vi "wavedump.vi"() -> ()   [LabVIEW 2018]
panel:
  in  "Plot":bool
  in  "?":enum32{"Output", "README"}(tab)
  out "Command Line Output":string
  in  "Stop":bool
  in  "Start":bool
  in  "Run":bool
  in  "Write":bool
  in  "Close":bool
  # "This vi is used to send wavedump commands.\n\nRun to run wavedump\n\nStart to start data aquisition\n\nWrite to start writing to file\n\nSTOP to stop data aquisition\n\nCLOSE to close the application."
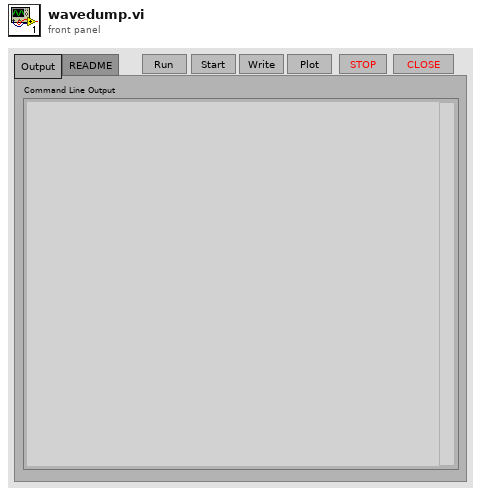
[diagram p1: front panel]
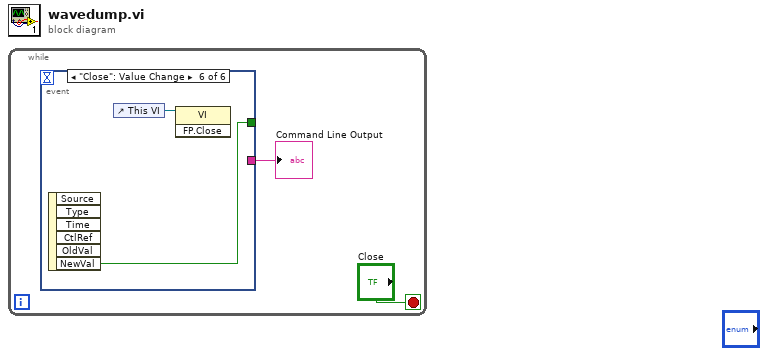
[diagram p0: block diagram]
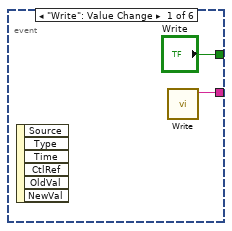
[diagram p2: hidden frame]
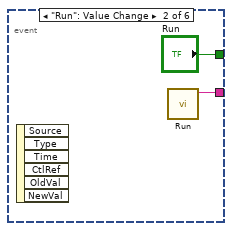
[diagram p3: hidden frame]
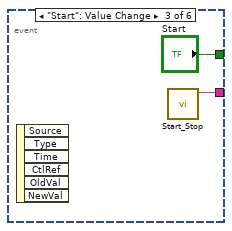
[diagram p4: hidden frame]
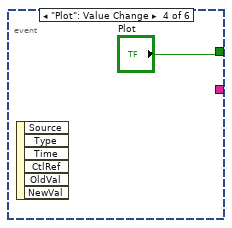
[diagram p5: hidden frame]
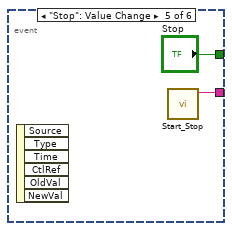
[diagram p6: hidden frame]
diagram:
  n1 = while {
    stop <- "Close" stop-if-true
    n2 = event shown="[5] \"Close\": Value Change" {
      selector: _ -> [_ _ _ _ _ _]
      dyn-events: _ -> [_ _ _ _ _ _]
      timeout: _ -> [_ _ _ _ _ _]
      tunnel: ["Write" "Run" "Start" "Plot" "Stop" w13] -> _
      tunnel: [w3 w5 w7 _ w10 _] -> w1
      event "Write": Value Change {
        n3 = event-data() -> ()  [unwired: 1 in, 6 out]
        n4 = call "Write.vi"() -> ("Command Line Output"=w3:string)  [unwired: 11 in]
      }
      event "Run": Value Change {
        n5 = event-data() -> ()  [unwired: 1 in, 6 out]
        n6 = call "Run.vi"() -> ("Command Line Output"=w5:string)  [unwired: 11 in]
      }
      event "Start": Value Change {
        n7 = event-data() -> ()  [unwired: 1 in, 6 out]
        n8 = call "Start_Stop.vi"() -> ("Command Line Output"=w7:string)  [unwired: 10 in]
      }
      event "Plot": Value Change {
        n9 = event-data() -> ()  [unwired: 1 in, 6 out]
      }
      event "Stop": Value Change {
        n10 = event-data() -> ()  [unwired: 1 in, 6 out]
        n11 = call "Start_Stop.vi"() -> ("Command Line Output"=w10:string)  [unwired: 10 in]
      }
      event "Close": Value Change {
        n12 = event-data() -> ("NewVal"=w13:bool)  [unwired: 1 in, 5 out]
        n13 = control-ref of="This VI"() -> (w12:refnum<vi>)
        n14 = invoke class="VI" method="FP.Close"(reference=w12) -> ()  [unwired: 2 in, 3 out]
      }
    }
    "Command Line Output" <- w1
  }
